vi "Save_to_Project.vi"(8 "error in (no error)":errorcluster, 9 "index":i32, 10 "buildObject":T1, 11 "AB_Source_RESTfulVI in":refnum<class "AB_Source_RESTfulVI.lvclass">) -> (0 "error out":errorcluster, 3 "AB_Source_RESTfulVI out":refnum<class "AB_Source_RESTfulVI.lvclass">)   [LabVIEW 2020, in "AB_Source_RESTfulVI.lvclass"]
uses:
  <vilib>/AppBuilder/AB_Classes/Source/RESTfulVI/AB_Source_RESTfulVI.lvclass
  <resource>/Framework/Providers/API/ItemRef.ctl
  <vilib>/AppBuilder/AB_Classes/Source/RESTfulVI/Configure_RESTfulVI/AB_RESTful_Configuration.ctl
  <vilib>/AppBuilder/AB_Classes/Source/RESTfulVI/Configure_RESTfulVI/AB_RESTful_VIType.ctl
  <vilib>/AppBuilder/AB_Classes/Source/RESTfulVI/Configure_RESTfulVI/AB_RESTful_OutputType.ctl
  <vilib>/AppBuilder/AB_Classes/Source/RESTfulVI/Configure_RESTfulVI/AB_RESTful_OutputFormat.ctl
  <vilib>/AppBuilder/AB_Classes/Source/RESTfulVI/AB_Source_RESTfulVI.lvclass/AB_Source_RESTfulVI.ctl
  <vilib>/AppBuilder/RW_Project/AB_RW_Project_Source_RESTfulVI_Data.ctl
  <vilib>/AppBuilder/RW_Project/AB_RW_Project_PropBag_Action.ctl
  <vilib>/AppBuilder/AB_Classes/Source/VI/AB_Source_VI.lvclass
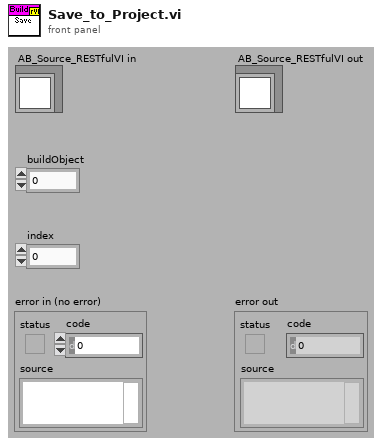
[diagram p1: front panel]
types:
  T1 = typedef "ItemRef.ctl" = u64
  T2 = typedef "AB_RESTful_Configuration.ctl" = cluster{"Service VI Type":T3, "Load VI at statup":bool, "Keep VI in memory":bool, "Output type":T4, "Output format":T5, "Use headers":bool, "Buffered":bool, "eng_Load VI by name":bool}
  T3 = typedef "AB_RESTful_VIType.ctl" = enum32{"Web Method", "Auxiliary", "eng_Internal", "eng_Content"}
  T4 = typedef "AB_RESTful_OutputType.ctl" = enum32{"Terminal", "Stream"}
  T5 = typedef "AB_RESTful_OutputFormat.ctl" = enum32{"XML", "Text", "HTML", "JSON"}
  T6 = typedef "AB_RW_Project_Source_RESTfulVI_Data.ctl" = cluster{"RESTful VI configuration":T2}
  T7 = typedef "AB_RW_Project_PropBag_Action.ctl" = enum16{"read", "write", "clear", "readPrevious", "writePrevious", "clearPrevious"}
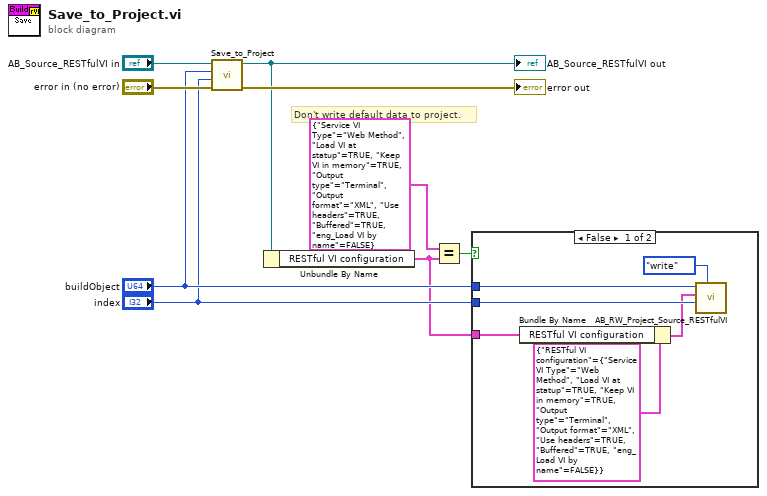
[diagram p0: block diagram]
diagram:
  # "Don't write default data to project."
  n1 = call-parent "Save_to_Project.vi"("error in (no error)"="error in (no error)", "index"="index", "buildObject"="buildObject", "AB_Source_VI in"="AB_Source_RESTfulVI in") -> ("error out"=→"error out":errorcluster, "AB_Source_VI out"=w4:refnum<class "AB_Source_RESTfulVI.lvclass">)  [unwired: 6 in]
  "AB_Source_RESTfulVI out" <- w4
  n2 = Unbundle By Name(w4) -> ("RESTful VI configuration"=w1:T2)
  n3 = Equal?(x=T2 {"Service VI Type"=enum."Web Method", "Load VI at statup"=TRUE, "Keep VI in memory"=TRUE, "Output type"=enum."Terminal", "Output format"=enum."XML", "Use headers"=TRUE, "Buffered"=TRUE, "eng_Load VI by name"=FALSE} ("RESTful VI configuration"), y=w1) -> (x = y?=w2:bool)
  n4 = case shown="False" w2 {
    tunnel: "buildObject" -> [w14 _]
    tunnel: "index" -> [w13 _]
    tunnel: w1 -> [w11 _]
    frame False {
      n5 = Bundle By Name(cluster=T6 {"RESTful VI configuration"={"Service VI Type"=enum."Web Method", "Load VI at statup"=TRUE, "Keep VI in memory"=TRUE, "Output type"=enum."Terminal", "Output format"=enum."XML", "Use headers"=TRUE, "Buffered"=TRUE, "eng_Load VI by name"=FALSE}} ("dataSource in"), "RESTful VI configuration"=w11) -> (w10:T6)
      n6 = call <vilib>:"AB_RW_Project_Source_RESTfulVI.vi"("action"=AB_RW_Project_PropBag_Action."write", "index in"=w13, "dataSource in"=w10, "buildObject"=w14) -> ()  [unwired: 4 in, 4 out]
    }
    frame True {
    }
  }
